vi "Close Demosaicker.vi"(8 "error in (no error)":errorcluster, 11 "Demosaicker reference":refnum<k24>) -> (0 "error out":errorcluster)   [LabVIEW 2020]
uses:
  C:/GEECS/Developers Version/source/Device Drivers/Point Grey Camera/Library_X86/Thorlabs.TSI.Demosaicker.dll
  Point Grey Camera/Library_X86/Thorlabs.TSI.Demosaicker.dll
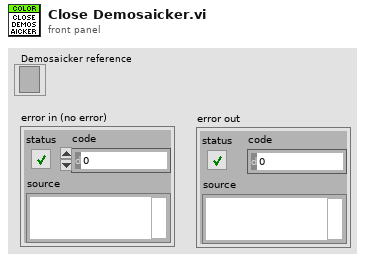
[diagram p1: front panel]
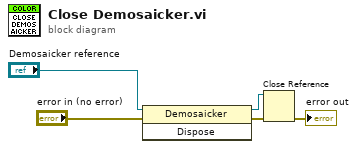
[diagram p0: block diagram]
diagram:
  n1 = invoke class="Demosaicker" method="Dispose"(reference="Demosaicker reference", error in="error in (no error)") -> (reference out=w3:refnum<k24>, error out=w4:errorcluster)  [unwired: 1 in, 1 out]
  n2 = Close Reference(reference=w3, error in (no error)=w4) -> (error out=→"error out":errorcluster)
